vi "Write ClockParameters.vi"(7 "ClockEnable":bool, 8 "error in (no error)":errorcluster, 9 "PrescalerCrystalOscilator":u32=8, 10 "ClockSource":T1=1 items=["Internal Oscillator"=1, "External Trigger"=2, "Trigger-> Oscillator"=3, "MasterSlave Bus"=4], 11 "BME_DG_Base in":refnum<class "BME_DG_Base.lvclass">) -> (0 "error out":errorcluster, 3 "BME_DG_Base out":refnum<class "BME_DG_Base.lvclass">)   [LabVIEW 2009, in "POLARIS BME DG.lvlib" / "BME_DG_Base.lvclass"]
uses:
  BME_DG_Base.lvclass
  LV-BME Interface/ClockSource.ctl
  BME_DG_Base.lvclass/BME_DG_Base.ctl
  POLARIS BME DG.lvlib
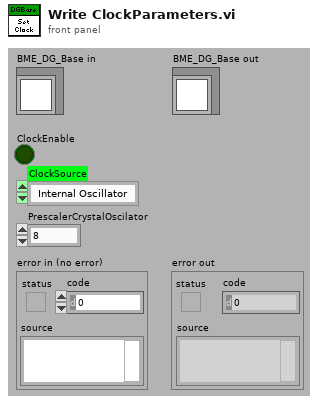
[diagram p1: front panel]
types:
  T1 = typedef "POLARIS BME DG.lvlib/ClockSource.ctl" = i32
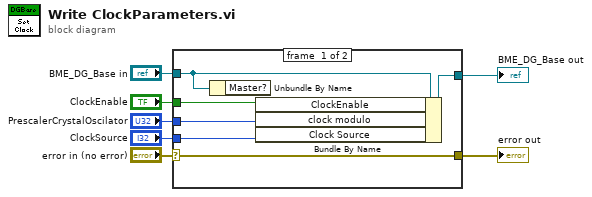
[diagram p0: block diagram]
diagram:
  n1 = case shown="No Error" "error in (no error)" {
    selector: "error in (no error)" -> [w13 w15]
    tunnel: [w13 w15] -> w6
    tunnel: [w12 w14] -> w4
    tunnel: "BME_DG_Base in" -> [w9 w14]
    tunnel: "ClockEnable" -> [w8 _]
    tunnel: "PrescalerCrystalOscilator" -> [w11 _]
    tunnel: "ClockSource" -> [w10 _]
    frame #0 {
      n2 = Unbundle By Name(w9) -> ()  [unwired: 1 out]
      n3 = Bundle By Name(cluster=w9, "ClockEnable"=w8, "clock modulo"=w11, "Clock Source"=w10) -> (w12:refnum<class "BME_DG_Base.lvclass">)
    }
    frame #1 {
    }
  }
  "error out" <- w6
  "BME_DG_Base out" <- w4
